vi "Hi_Port_Test.vi"(0 "datain":string[](array[string])=["备注", "负载通道", "负载地址", "延时时间", "output max", "output min", "量测类型", "待测物板号"], 5 "HW CH Number":i32=4, 7 "Setup":string) -> (4 "REPORT INDECATE":string[][](array[string])=[["微安测试", "", "", "", ""], ["微安量测", "4", "0.000", "0.1", "NG"], ["微安量测", "4", "0.000", "0.1", "NG"], ["微安量测", "4", "0.000", "0.1", "NG"], ["微安量测", "4", "0.000", "0.1", "NG"]], 6 "ROW HEAD":string[](array[string]), 8 "PF":string[](array[string]), 10 "testData":string[](array[string]), 14 "数组":bool[](array[boolean]), 15 "Array":string[](array[string]))   [LabVIEW 2018]
uses:
  Subvi/Global.vi
panel:
  out "测试板数":i32=4
  # "[VoltageTest]\nExt.Name =2222222222;\nAddress =1;\nDelay Time =1;\nMAX.Spec =*;\nMin.Spec =2;\nTest Type =;\nRelayH_8Bit =0,0,0,0;\nRelayL_8Bit =0,0,0,0;\nStart board number =1;#"
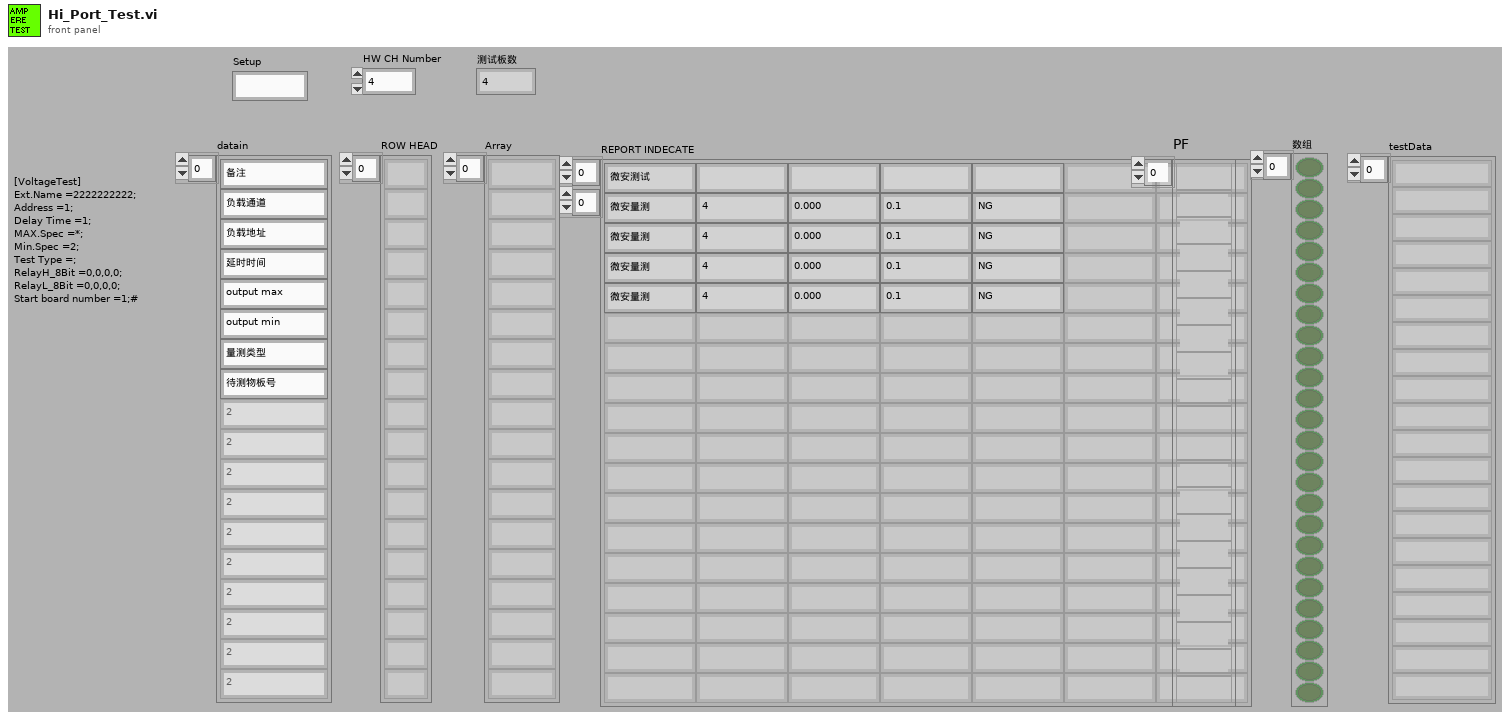
[diagram p1: front panel]
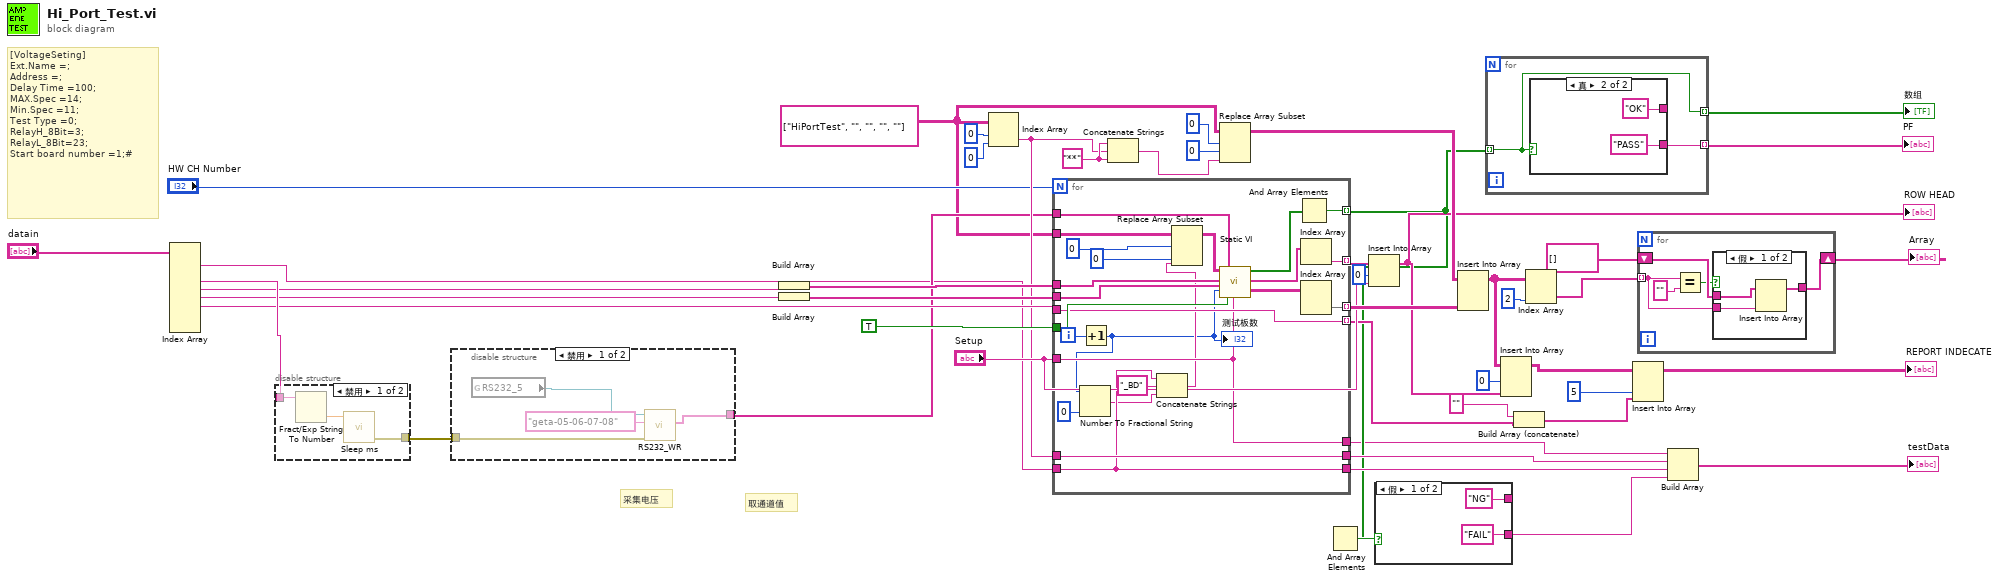
[diagram p0: block diagram]
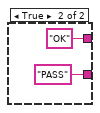
[diagram p4: hidden frame]
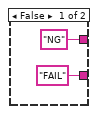
[diagram p5: hidden frame]
diagram:
  w1 = string[][] [["HiPortTest", "", "", "", ""]]
  w38 = "**" ("字符串")
  # "取通道值"
  # "采集电压"
  # "[VoltageSeting]\nExt.Name =;\nAddress =;\nDelay Time =100;\nMAX.Spec =14;\nMin.Spec =11;\nTest Type =0;\nRelayH_8Bit=3;\nRelayL_8Bit=23;\nStart board number =1;#"
  n1 = Index Array(array="datain") -> (element #1=w2:string, element #3=w41:string, element #4=w34:string, element #5=w33:string, element #6=w21:string)  [unwired: 9 in, 4 out]
  n2 = disable-structure shown="禁用" {
    disable-tunnel: w41 -> [w50 _]
    disable-tunnel: [w49 _] -> w5
    frame Disabled {
      n3 = Fract/Exp String To Number(string=w50) -> (number=w48:dbl)  [unwired: 3 in, 1 out]
      n4 = call "Sleep ms.vi"("等待时间（毫秒）"=w48) -> ("error out"=w49:errorcluster)  [unwired: 10 in]
    }
    frame Enabled {
    }
  }
  n5 = disable-structure shown="禁用" {
    disable-tunnel: w5 -> [w53 _]
    disable-tunnel: [w51 _] -> w3
    frame Disabled {
      n6 = global read "Global.vi" "RS232_5"() -> (w52:refnum<visa-resource-name>)
      n7 = call "RS232_WR.vi"("error in (no error)"=w53, "CMD"="geta-05-06-07-08", "VISA资源名称"=w52) -> ("Out data"=w51:string[])  [unwired: 6 in, 2 out]
    }
    frame Enabled {
    }
  }
  n8 = Build Array(w34) -> (w32:string[])
  n9 = Build Array(w33) -> (w31:string[])
  n10 = Index Array(array=w1, index (row)=0 ("索引 (行)"), index (col)=0 ("禁用的索引 (列)")) -> (element=w14:string)
  n11 = for {
    N: "HW CH Number" -> [_]
    tunnel: w3 -> [w78]
    tunnel: w32 -> [w77]
    tunnel: w31 -> [w76]
    tunnel: "Setup" -> [w66]
    tunnel: TRUE -> [w74]
    tunnel: [w73] -> w10 mode=indexing
    tunnel: [w71] -> w27 mode=indexing
    tunnel: [w69] -> w28 mode=indexing
    tunnel: w21 -> [w68]
    tunnel: [w68] -> w17 mode=indexing
    tunnel: w14 -> [w67]
    tunnel: [w67] -> w13
    tunnel: w2 -> [w58]
    tunnel: [w58] -> w12
    tunnel: [w66] -> w7
    tunnel: w1 -> [w64]
    i -> [w61]
    n12 = Increment(x=w61) -> (x+1=w55:i32)
    "测试板数" <- w55
    n13 = Number To Fractional String(number=w55, precision (6)=i16 0 ("精度(6)")) -> (F-format string=w57:string)  [unwired: 2 in]
    n14 = Concatenate Strings(w58, "_BD" ("字符串"), w57) -> (w56:string)
    n15 = Replace Array Subset(array=w64, new element=w56, index (row)=0 ("索引 (行)"), index (col)=0 ("禁用的索引 (列)")) -> (w63:string[][])
    n16 = call "Static VI.vi"("添加的数组"=w63, "Max"=w77, "Min"=w76, "板数"=w55, "INPUTSTRING"=w78, "是否为字符串对比"=w74, "SQ"=w66) -> ("P/F"=w75:bool[], "SQ out"=w72:string[], "arrauy out"=w70:string[][])  [unwired: 9 in, 1 out]
    n17 = And Array Elements(Boolean array=w75) -> (logical AND=w73:bool)
    n18 = Index Array(array=w72) -> (element=w71:string)  [unwired: 1 in]
    n19 = Index Array(array=w70) -> (element=w69:string[])  [unwired: 2 in]
  }
  n20 = Concatenate Strings(w38, w14, w38) -> (w35:string)
  n21 = Replace Array Subset(array=w1, new element=w35, index (row)=0 ("索引 (行)"), index (col)=0 ("禁用的索引 (列)")) -> (w29:string[][])
  n22 = And Array Elements(Boolean array=w10) -> (logical AND=w11:bool)
  n23 = Insert Into Array(array=w27, index=0 ("索引"), new element="Setup") -> (w23:string[])
  "ROW HEAD" <- w23
  n24 = case shown="假" w11 {
    tunnel: ["NG" "OK"] -> _
    tunnel: ["FAIL" "PASS"] -> w9
    frame False {
    }
    frame True {
    }
  }
  n25 = Insert Into Array ("数组插入")(array=w29, new element=w28) -> (w24:string[][])  [unwired: 2 in]
  n26 = for {
    tunnel: w10 -> [w83] mode=indexing
    tunnel: [w84] -> w43 mode=indexing
    tunnel: [w83] -> w6 mode=indexing
    n27 = case shown="真" w83 {
      tunnel: ["NG" "OK"] -> _
      tunnel: ["FAIL" "PASS"] -> w84
      frame False {
      }
      frame True {
      }
    }
  }
  "PF" <- w43
  "数组" <- w6
  n28 = Insert Into Array(array=w24, index (col)=0 ("禁用的索引 (列)"), new element=w23) -> (w19:string[][])  [unwired: 1 in]
  n29 = Build Array (concatenate)("" ("字符串"), w17) -> (w15:string[])
  n30 = Index Array(array=w24, index (col)=2 ("禁用的索引 (列)")) -> (element=w45:string[])  [unwired: 1 in]
  n31 = Insert Into Array(array=w19, index (col)=5 ("禁用的索引 (列)"), new element=w15) -> (→"REPORT INDECATE":string[][])  [unwired: 1 in]
  n32 = for {
    tunnel: w45 -> [w89] mode=indexing
    shift-right: [w90] -> w44
    shift-left: string[] [] ("Array") -> [w93]
    n33 = Equal?(x=w89, y="") -> (x = y?=w91:bool)
    n34 = case shown="假" w91 {
      tunnel: w93 -> [w96 w97]
      tunnel: [w95 w97] -> w90
      tunnel: w89 -> [w94 _]
      frame False {
        n35 = Insert Into Array(array=w96, new element=w94) -> (w95:string[])  [unwired: 1 in]
      }
      frame True {
      }
    }
  }
  "Array" <- w44
  n36 = Build Array(w7, w13, w12, w9) -> (→"testData":string[])
